vi "RFmx_Cntr_Configure.vi"(7 "Meas_Type":string[](array[string])=["ACP"], 8 "error in (no error)":errorcluster, 10 "RFmx_Parameters":T1={"Default"={"Center_Freq(Hz)"=1150000000.0, "Ref_Level(dBm)"=-10.0, "Span(Hz)"=20000000.0, "RBW(Hz)"=10000.0, "RBW Filter Type"=enum."Gaussian", "Ch_IBW(Hz)"=3840000.0, "Sweep_Time(s)"=0.01, "Num_of_Average"=0, "IQ_Bandwidth(Hz)"=20000000.0}, "ACP_Offset_Freq"=[5000000.0, 10000000.0, 12500000.0], "ACP_Offset_IBW"=[3840000.0, 3840000.0, 3840000.0], "OBW_Percent(%)"=95.0, "TXP_Interval(s)"=0.01, "CCDF_Interval(s)"=0.01, "CCDF_Threshold"=20000000.0, "SFDR_Span(Hz)"=20000000.0, "Harms_RBW(Hz)"=10000.0, "Harms_RBW_Filter"=enum."Gaussian"} {"Harms_RBW(Hz)" format="%.3p"; "TXP_Interval(s)" format="%#_6p"; "SFDR_Span(Hz)" format="%#_6p"; "CCDF_Threshold" format="%#_6p"; "CCDF_Interval(s)" format="%#_6p"; "OBW_Percent(%)" format="%#_6p"; "ACP_Offset_IBW" format="%#_6p"; "ACP_Offset_Freq" format="%#_6p"; "Default"."IQ_Bandwidth(Hz)" format="%#_6p"; "Default"."Num_of_Average" format="%#_6p"; "Default"."Sweep_Time(s)" format="%#_6p"; "Default"."Ch_IBW(Hz)" format="%.3p"; "Default"."RBW(Hz)" format="%.3p"; "Default"."Span(Hz)" format="%.3p"; "Default"."Ref_Level(dBm)" format="%.3p"; "Default"."Center_Freq(Hz)" format="%.3p"}, 11 "Instrument Handle in":refnum<k21>="VST") -> (0 "error out":errorcluster, 3 "Instrument Handle out":refnum<k21>="VST")   [LabVIEW 2014]
uses:
  15_DataManagement/Config_RFmx_Settings.ctl
  <vilib>/RFmx/RFInstr/mx/RFmxInstr.llb/RFmxInstr Build Signal String.vi
  <vilib>/RFmx/SpecAn/mx/RFmxSpecAn.llb/RFmxSpecAn Select Measurement (Single).vi
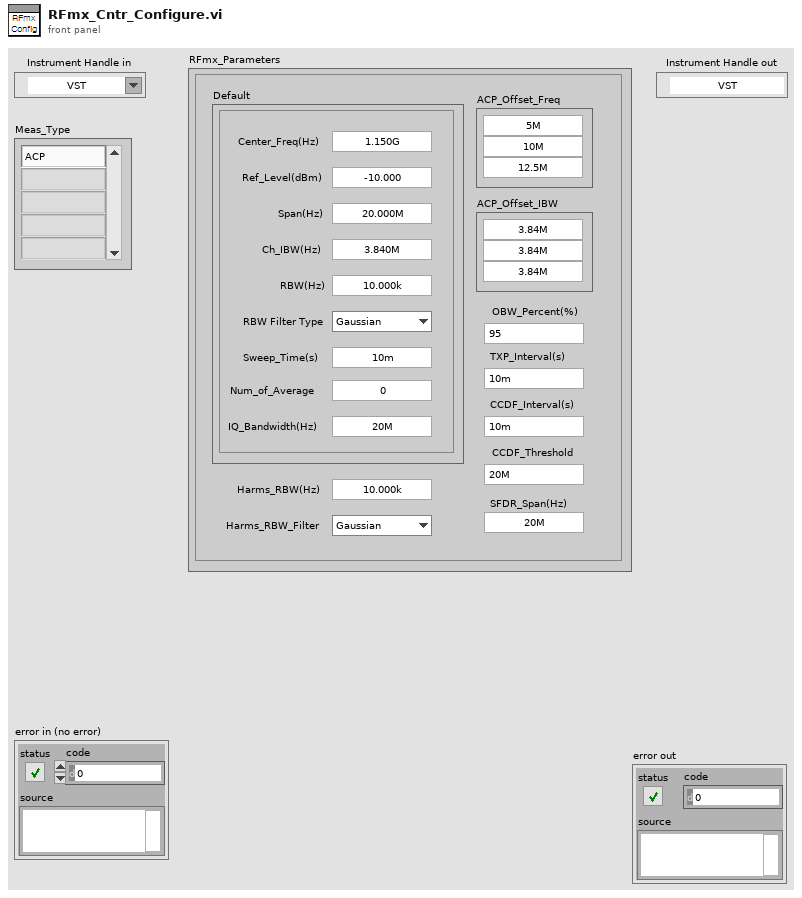
[diagram p1: front panel]
types:
  T1 = typedef "Config_RFmx_Settings.ctl" = cluster{"Default":cluster{"Center_Freq(Hz)":dbl, "Ref_Level(dBm)":dbl, "Span(Hz)":dbl, "RBW(Hz)":dbl, "RBW Filter Type":enum16{"FFT Based", "Gaussian", "Flat", "Synch Tuned - 4", "Synch Tuned - 5"}, "Ch_IBW(Hz)":dbl, "Sweep_Time(s)":dbl, "Num_of_Average":i32, "IQ_Bandwidth(Hz)":dbl}, "ACP_Offset_Freq":dbl[], "ACP_Offset_IBW":dbl[], "OBW_Percent(%)":dbl, "TXP_Interval(s)":dbl, "CCDF_Interval(s)":dbl, "CCDF_Threshold":dbl, "SFDR_Span(Hz)":dbl, "Harms_RBW(Hz)":dbl, "Harms_RBW_Filter":enum16{"FFT Based", "Gaussian", "Flat", "Synch Tuned - 4", "Synch Tuned - 5"}}
  T2 = enum16{"ACP", "CCDF", "CHP", "FCnt", "Harmonics", "OBW", "SEM", "Spectrum", "Spur", "TXP", "AMPM", "DPD", "IQ"}
  T3 = enum16{"FFT Based", "Gaussian", "Flat", "Synch Tuned - 4", "Synch Tuned - 5"}
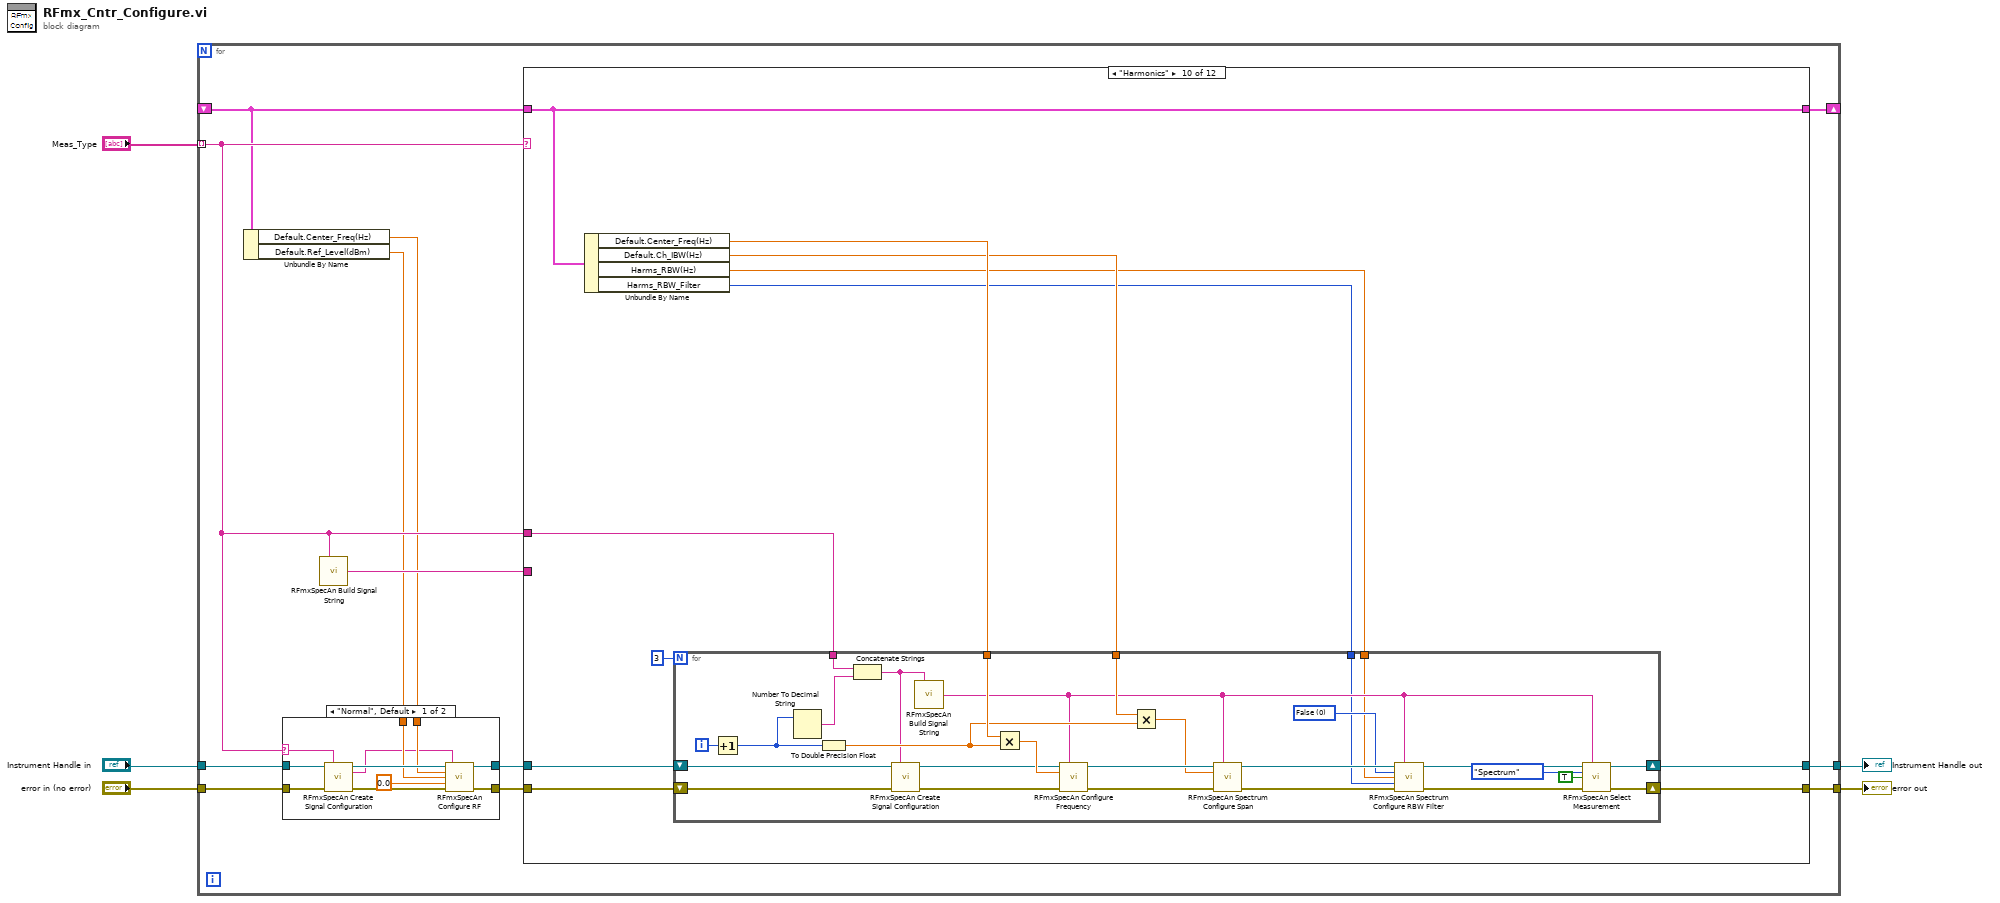
[diagram p0: block diagram]
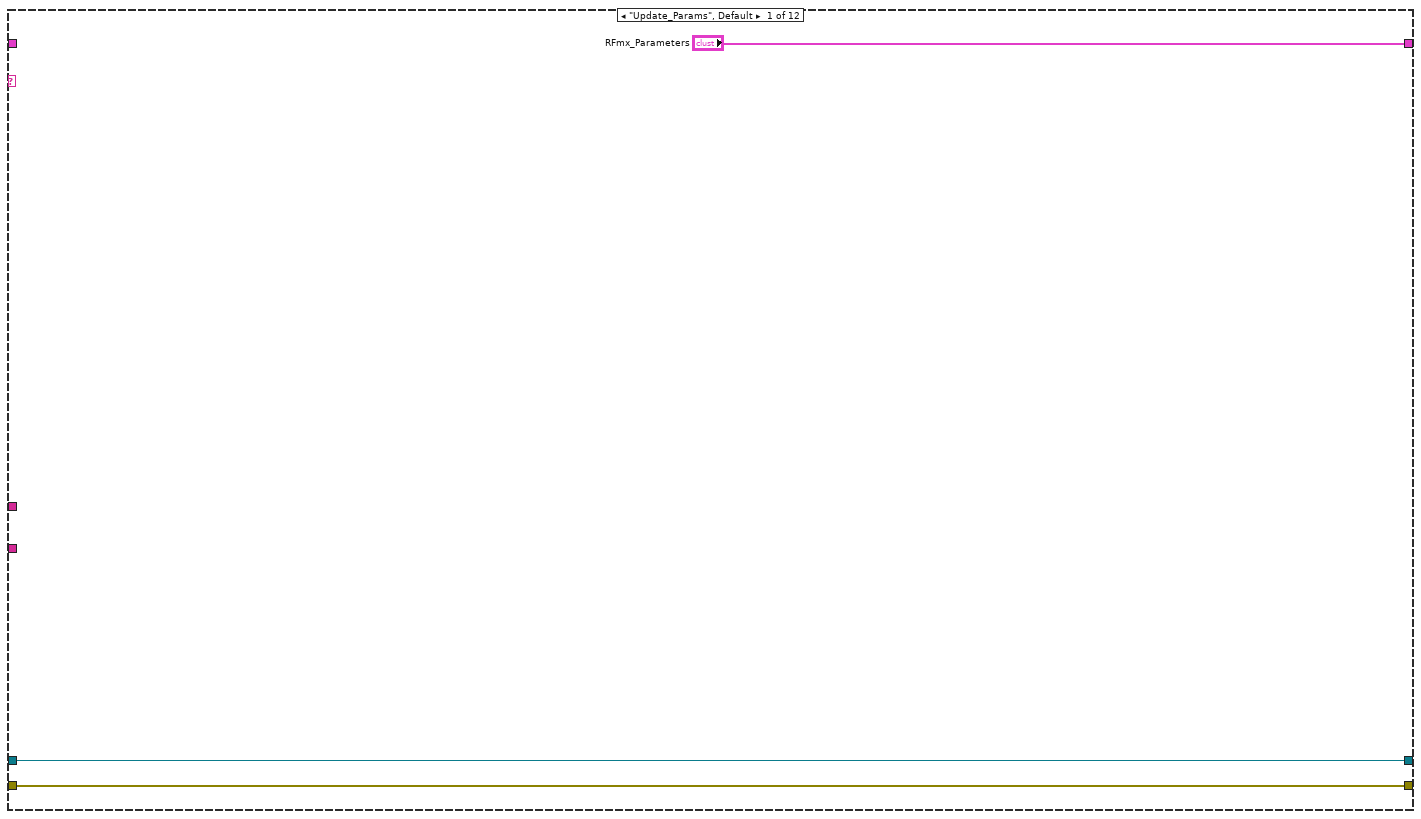
[diagram p3: hidden frame]
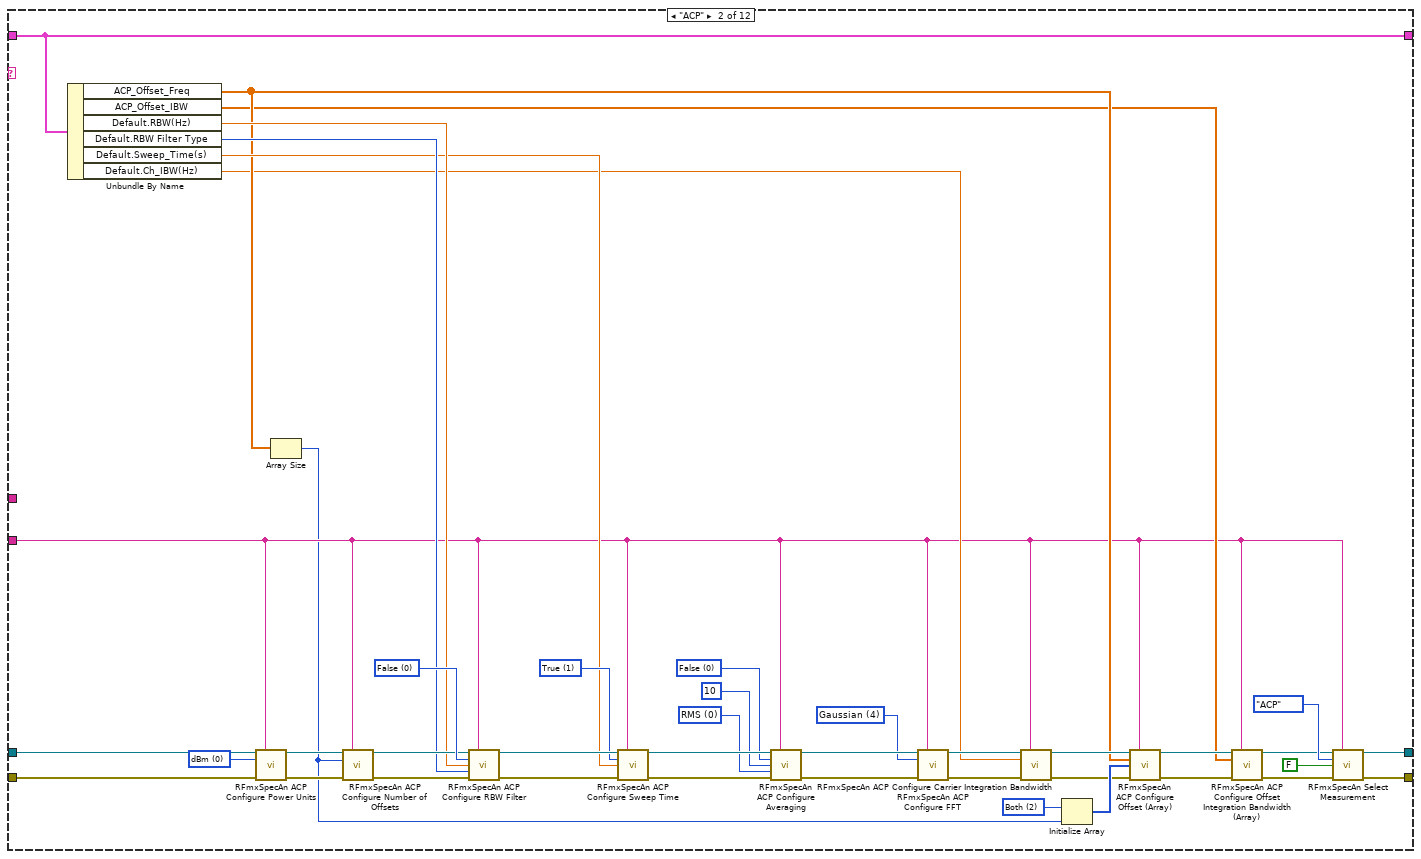
[diagram p4: hidden frame]
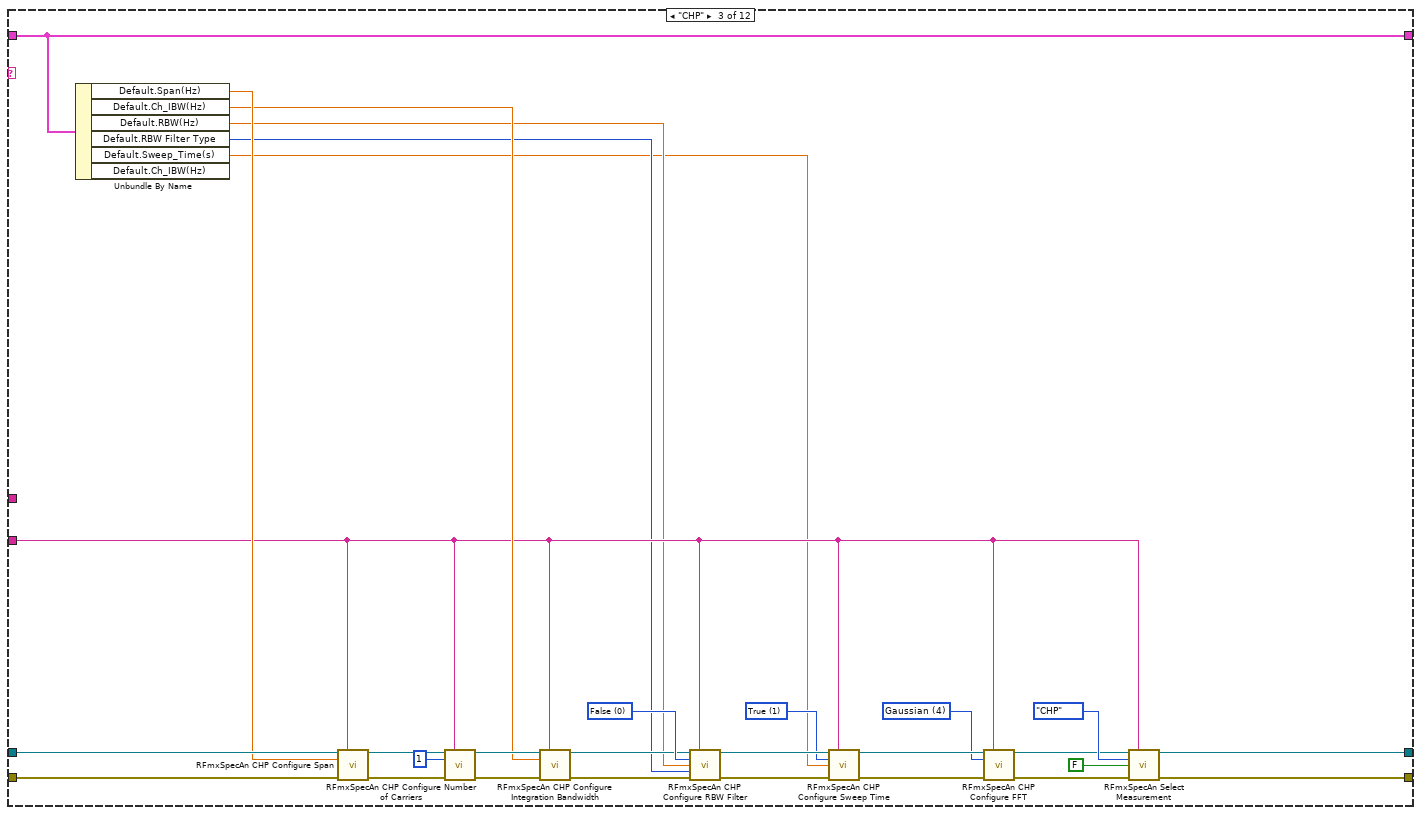
[diagram p5: hidden frame]
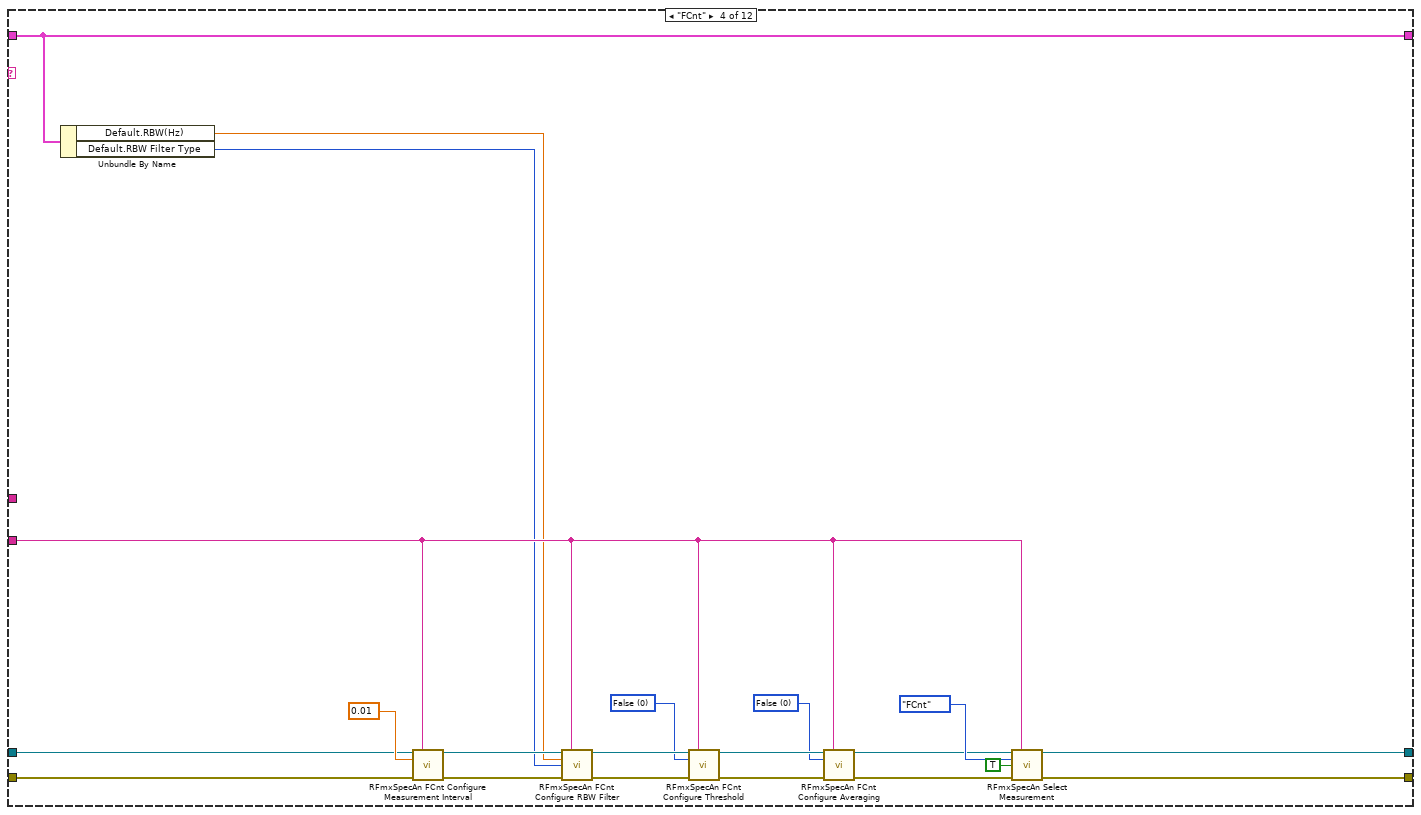
[diagram p6: hidden frame]
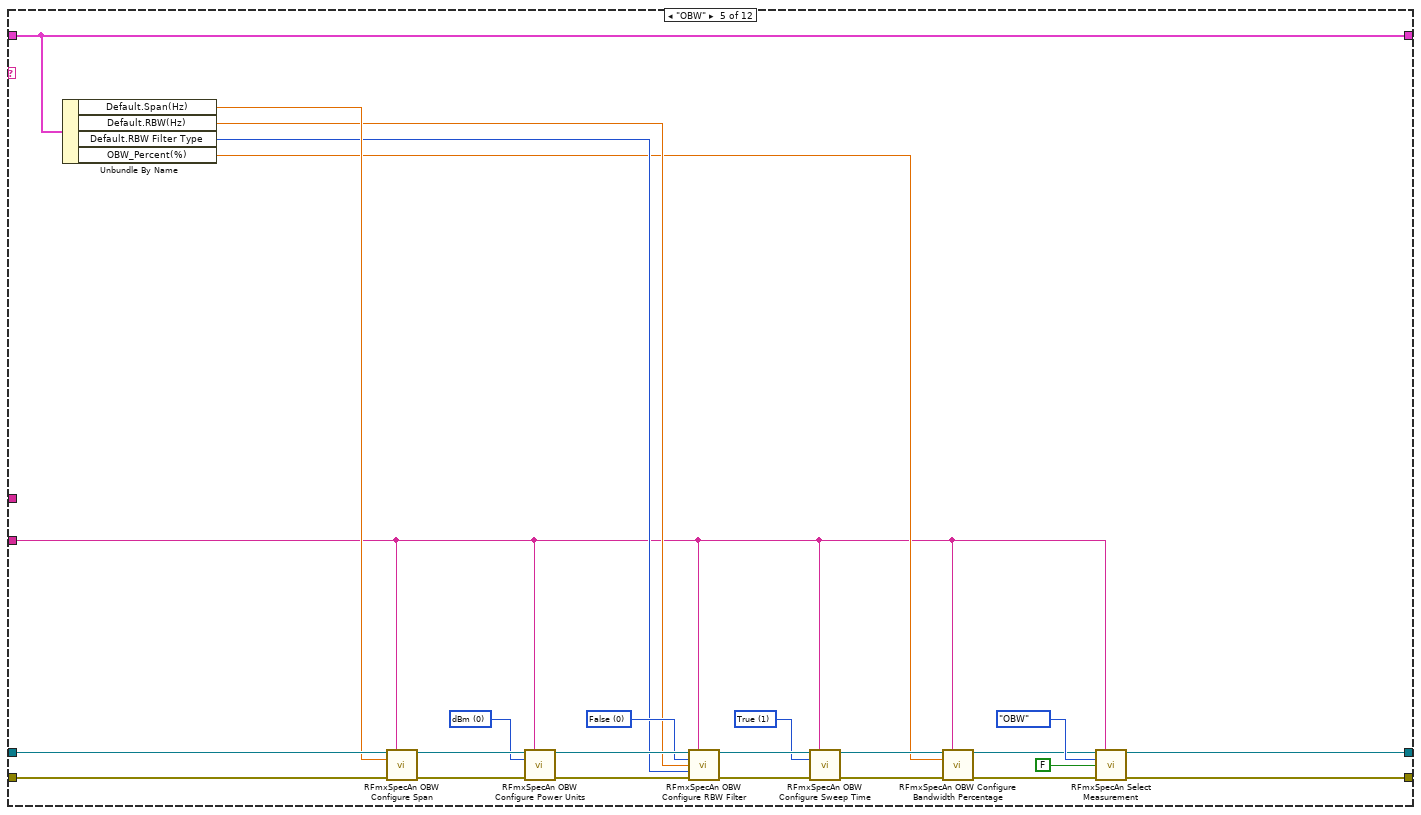
[diagram p7: hidden frame]
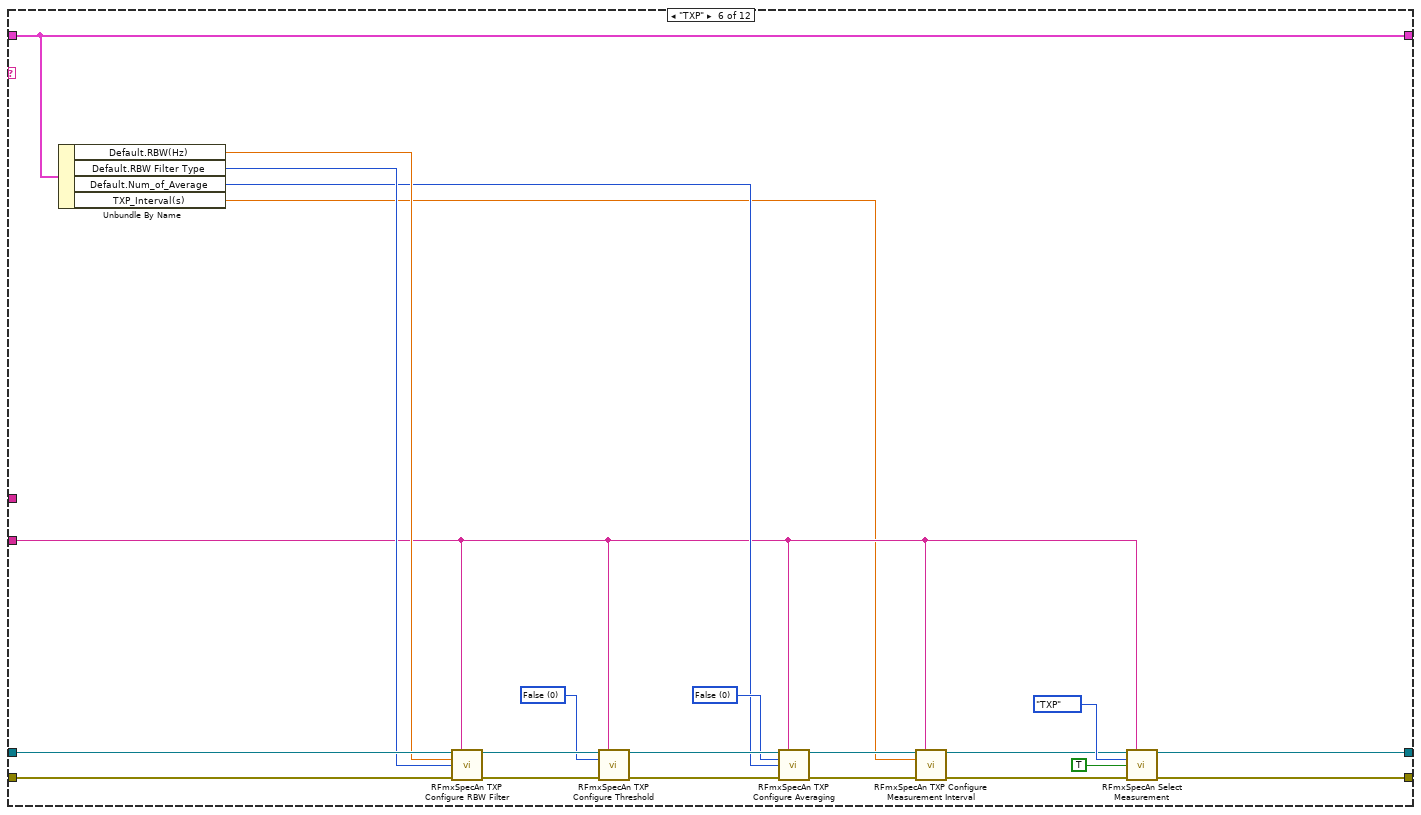
[diagram p8: hidden frame]
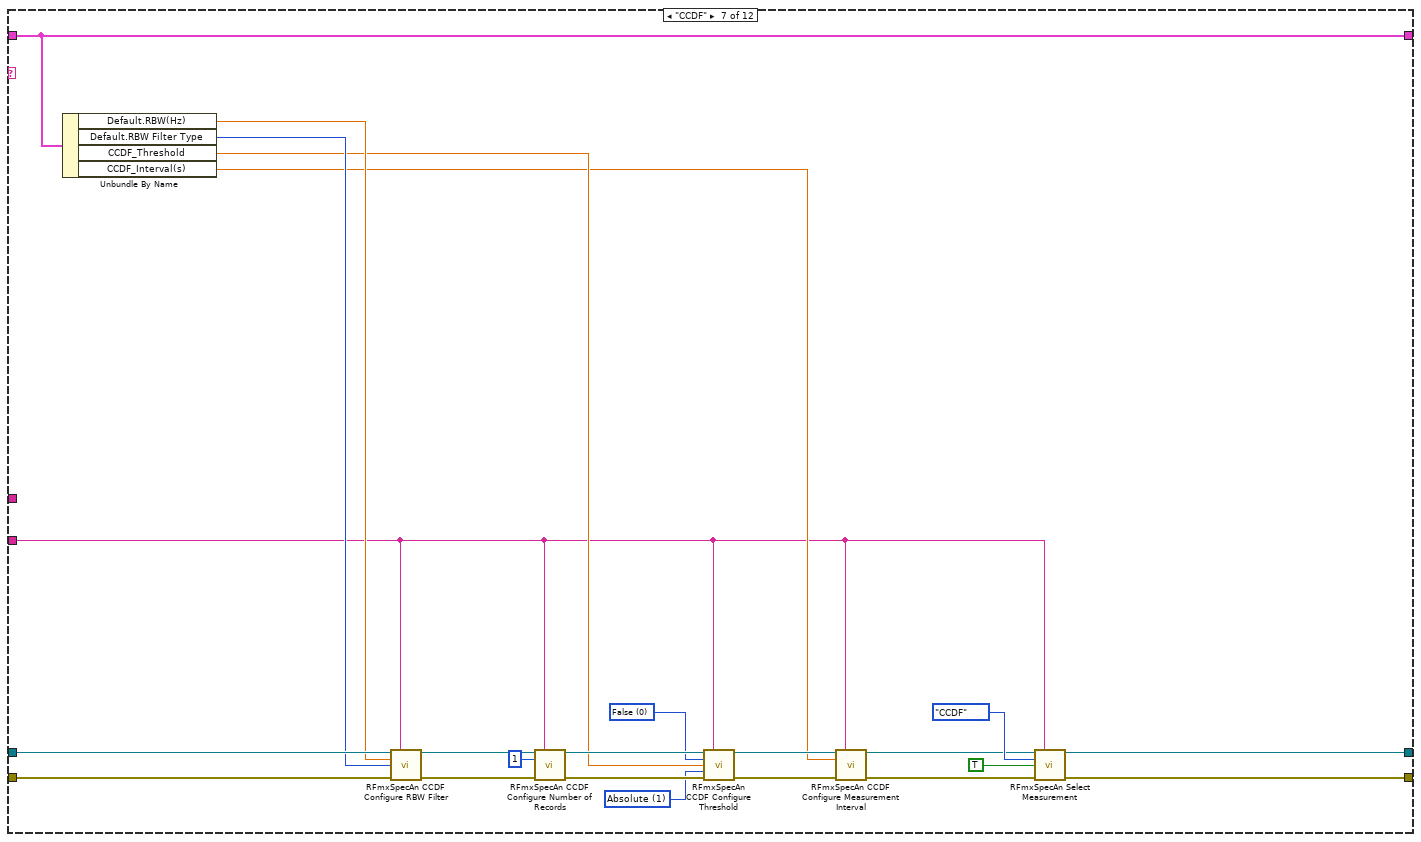
[diagram p9: hidden frame]
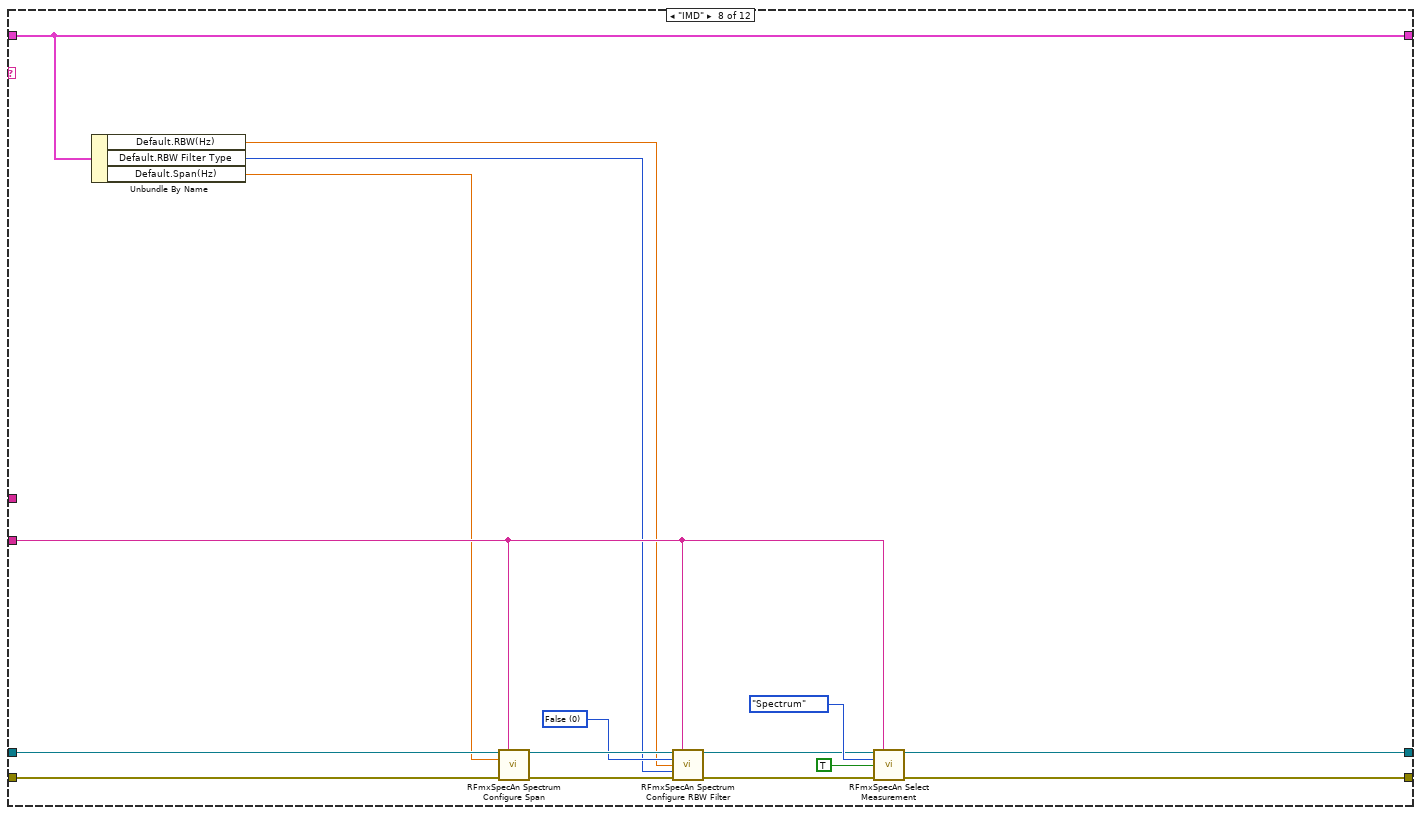
[diagram p10: hidden frame]
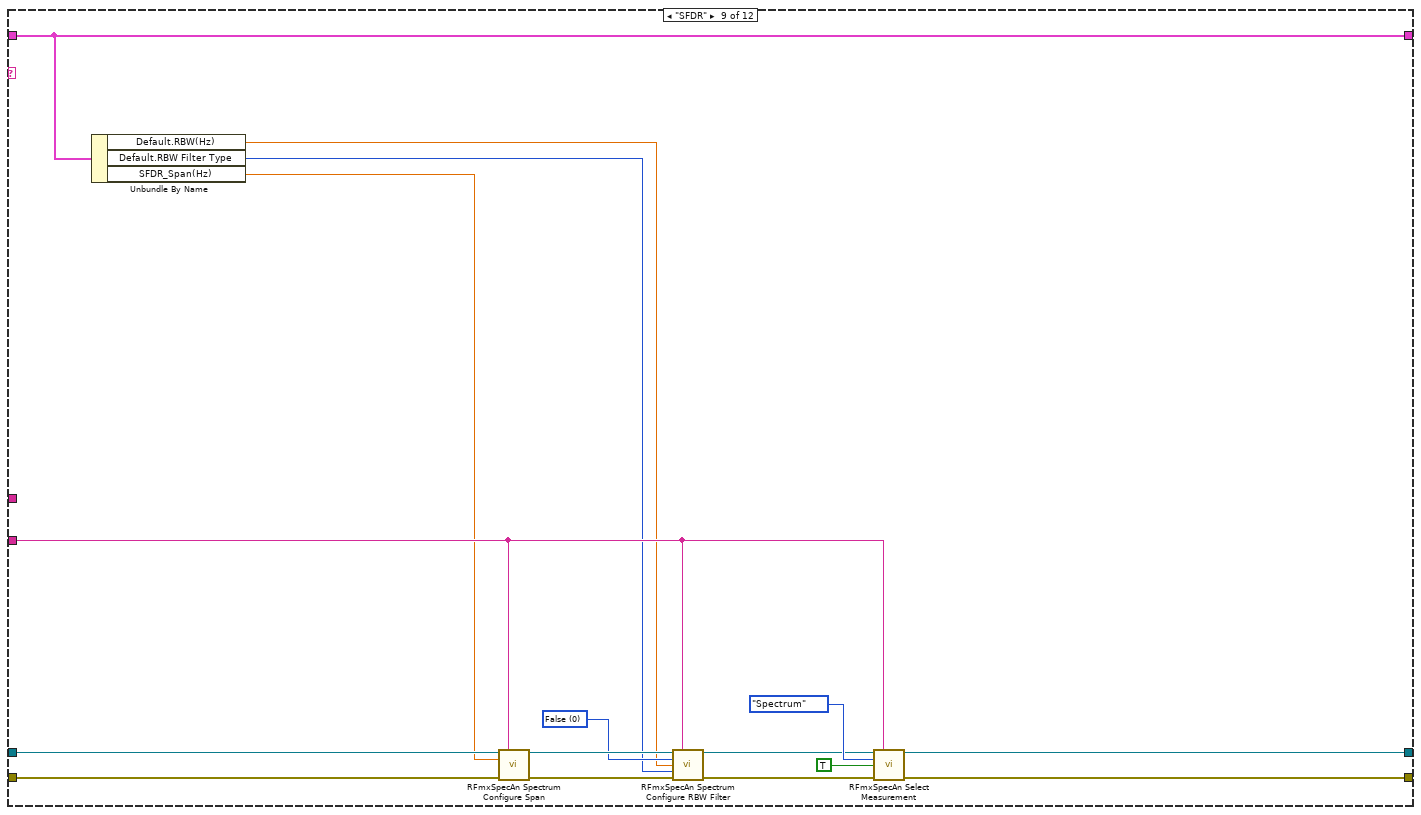
[diagram p11: hidden frame]
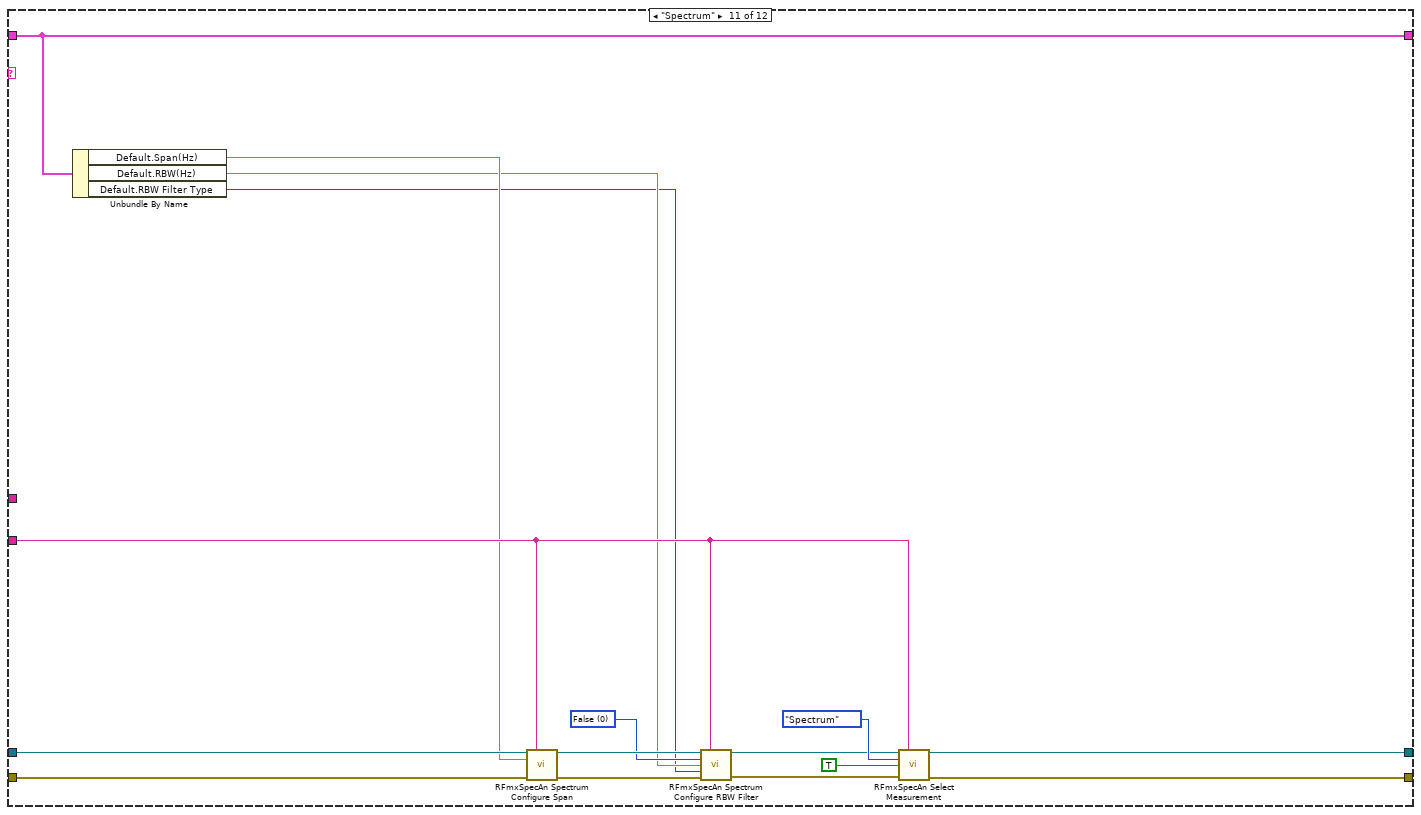
[diagram p12: hidden frame]
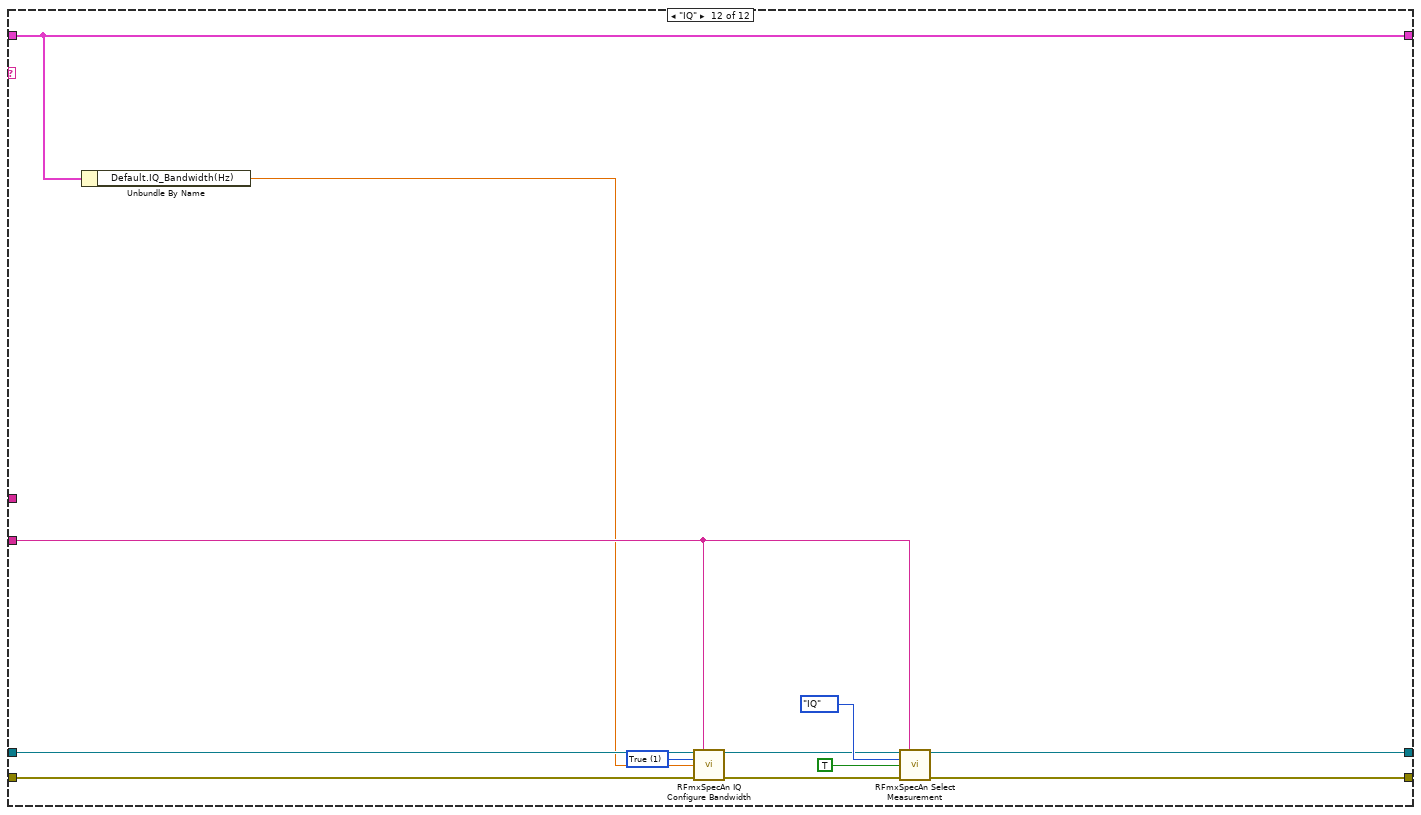
[diagram p13: hidden frame]
diagram:
  n1 = for {
    tunnel: [w17] -> w5
    tunnel: [w16] -> w4
    tunnel: "Meas_Type" -> [w13] mode=indexing
    tunnel: "Instrument Handle in" -> [w15]
    tunnel: "error in (no error)" -> [w14]
    shift-right: [w9] -> _
    shift-left: _ -> [w8]
    n2 = Unbundle By Name(w8) -> ("Default.Center_Freq(Hz)"=w7:dbl, "Default.Ref_Level(dBm)"=w6:dbl)
    n3 = case shown="\"Normal\", Default" w13 {
      selector: w13 -> [w19 _]
      tunnel: w15 -> [w28 w30]
      tunnel: w14 -> [w27 w29]
      tunnel: [w24 w30] -> w11
      tunnel: [w23 w29] -> w10
      tunnel: w6 -> [w21 _]
      tunnel: w7 -> [w20 _]
      frame "Normal", Default {
        n4 = call <vilib>:"RFmxSpecAn Create Signal Configuration.vi"("Instrument Handle In"=w28, "Signal Name"=w19, "error in (no error)"=w27) -> ("Instrument Handle Out"=w25:refnum<k21>, "Selector String Out"=w18:string, "error out"=w22:errorcluster)  [unwired: 10 in]
        n5 = call <vilib>:"RFmxSpecAn Configure RF.vi"("Instrument Handle In"=w25, "Selector String"=w18, "Center Frequency (Hz)"=w20, "Reference Level (dBm)"=w21, "External Attenuation (dB)"=0.0, "error in (no error)"=w22) -> ("Instrument Handle Out"=w24:refnum<k21>, "error out"=w23:errorcluster)  [unwired: 8 in]
      }
      frame "Harmonics" {
      }
    }
    n6 = call <vilib>:"RFmxSpecAn Build Signal String.vi"("Signal Name"=w13) -> ("Selector String"=w12:string)  [unwired: 14 in]
    n7 = case shown="\"Harmonics\"" w13 {
      tunnel: w11 -> [w32 w58 w96 w116 w141 w166 w195 w205 w221 w237 w279 w293]
      tunnel: w10 -> [w31 w57 w95 w115 w140 w165 w194 w204 w220 w236 w278 w292]
      tunnel: [w32 w55 w89 w110 w138 w163 w185 w203 w219 w235 w274 w287] -> w16
      tunnel: [w31 w54 w88 w109 w137 w162 w184 w202 w218 w234 w273 w286] -> w17
      tunnel: w12 -> [_ w36 w81 w111 w128 w152 w173 w201 w217 _ w272 w288]
      tunnel: w13 -> [_ _ _ _ _ _ _ _ _ w233 _ _]
      tunnel: ["RFmx_Parameters" w34 w76 w107 w126 w158 w182 w200 w216 w228 w270 w283] -> w9
      tunnel: w8 -> [_ w34 w76 w107 w126 w158 w182 w200 w216 w228 w270 w283]
      frame "Update_Params", Default {
      }
      frame "ACP" {
        w48 = 2 items=["Neg", "Pos", "Both"] ("Offset Frequency Sideband")
        w63 = 1 items=["False", "True"] ("Sweep Time Auto")
        w64 = 0 items=["RMS", "Log", "Scalar", "Max", "Min", "Vector"] ("Averaging Type")
        w66 = 0 items=["False", "True"] ("Averaging Enabled")
        w67 = 4 items=["None", "Flat Top", "Hanning", "Hamming", "Gaussian", "Blackman", "Blackman-Harris", "Kaiser-Bessel"] ("FFT Window")
        w74 = 0 items=["False", "True"] ("RBW Auto")
        w75 = 0 items=["dBm", "dBm/Hz"] ("Power Units")
        n8 = Unbundle By Name(w34) -> ("ACP_Offset_Freq"=w41:dbl[], "ACP_Offset_IBW"=w39:dbl[], "Default.RBW(Hz)"=w52:dbl, "Default.RBW Filter Type"=w51:T3, "Default.Sweep_Time(s)"=w50:dbl, "Default.Ch_IBW(Hz)"=w40:dbl)
        n9 = call <vilib>:"RFmxSpecAn ACP Configure Power Units.vi"("Instrument Handle In"=w58, "Selector String"=w36, "Power Units"=w75, "error in (no error)"=w57) -> ("Instrument Handle Out"=w62:refnum<k21>, "error out"=w61:errorcluster)  [unwired: 10 in]
        n10 = Array Size(array=w41) -> (size(s)=w35:i32)
        n11 = call <vilib>:"RFmxSpecAn ACP Configure Number of Offsets.vi"("Instrument Handle In"=w62, "Selector String"=w36, "Number of Offsets"=w35, "error in (no error)"=w61) -> ("Instrument Handle Out"=w60:refnum<k21>, "error out"=w59:errorcluster)  [unwired: 10 in]
        n12 = call <vilib>:"RFmxSpecAn ACP Configure RBW Filter.vi"("Instrument Handle In"=w60, "Selector String"=w36, "RBW Auto"=w74, "RBW (Hz)"=w52, "RBW Filter Type"=w51, "error in (no error)"=w59) -> ("Instrument Handle Out"=w73:refnum<k21>, "error out"=w72:errorcluster)  [unwired: 8 in]
        n13 = call <vilib>:"RFmxSpecAn ACP Configure Sweep Time.vi"("Instrument Handle In"=w73, "Selector String"=w36, "Sweep Time Auto"=w63, "Sweep Time Interval (s)"=w50, "error in (no error)"=w72) -> ("Instrument Handle Out"=w71:refnum<k21>, "error out"=w70:errorcluster)  [unwired: 9 in]
        n14 = call <vilib>:"RFmxSpecAn ACP Configure Averaging.vi"("Instrument Handle In"=w71, "Selector String"=w36, "Averaging Enabled"=w66, "Averaging Count"=10, "Averaging Type"=w64, "error in (no error)"=w70) -> ("Instrument Handle Out"=w69:refnum<k21>, "error out"=w68:errorcluster)  [unwired: 8 in]
        n15 = call <vilib>:"RFmxSpecAn ACP Configure FFT.vi"("Instrument Handle In"=w69, "Selector String"=w36, "FFT Window"=w67, "error in (no error)"=w68) -> ("Instrument Handle Out"=w43:refnum<k21>, "error out"=w42:errorcluster)  [unwired: 10 in]
        n16 = call <vilib>:"RFmxSpecAn ACP Configure Carrier Integration Bandwidth.vi"("Instrument Handle In"=w43, "Selector String"=w36, "Integration Bandwidth (Hz)"=w40, "error in (no error)"=w42) -> ("Instrument Handle Out"=w45:refnum<k21>, "error out"=w44:errorcluster)  [unwired: 10 in]
        n17 = Initialize Array(w48, w35) -> (w49:i32[])
        n18 = call <vilib>:"RFmxSpecAn ACP Configure Offset (Array).vi"("Instrument Handle In"=w45, "Selector String"=w36, "Offset Frequency (Hz)"=w41, "Offset Sideband"=w49, "error in (no error)"=w44) -> ("Instrument Handle Out"=w46:refnum<k21>, "error out"=w47:errorcluster)  [unwired: 9 in]
        n19 = call <vilib>:"RFmxSpecAn ACP Configure Offset Integration Bandwidth (Array).vi"("Instrument Handle In"=w46, "Selector String"=w36, "Integration Bandwidth (Hz)"=w39, "error in (no error)"=w47) -> ("Instrument Handle Out"=w38:refnum<k21>, "error out"=w37:errorcluster)  [unwired: 10 in]
        n20 = call-poly <vilib>:"RFmxSpecAn Select Measurement.vi"("Instrument Handle In"=w38, "Selector String"=w36, "Measurement"=T2."ACP", "Enable All Traces"=FALSE, "error in (no error)"=w37) -> ("Instrument Handle Out"=w55:refnum<k21>, "error out"=w54:errorcluster)  [unwired: 9 in]
      }
      frame "CHP" {
        w97 = 4 items=["None", "Flat Top", "Hanning", "Hamming", "Gaussian", "Blackman", "Blackman-Harris", "Kaiser-Bessel"] ("FFT Window")
        w100 = 1 items=["False", "True"] ("Sweep Time Auto")
        w103 = 0 items=["False", "True"] ("RBW Auto")
        n21 = Unbundle By Name(w76) -> ("Default.Span(Hz)"=w85:dbl, "Default.Ch_IBW(Hz)"=w84:dbl, "Default.RBW(Hz)"=w80:dbl, "Default.RBW Filter Type"=w79:T3, "Default.Sweep_Time(s)"=w78:dbl)  [unwired: 1 out]
        n22 = call <vilib>:"RFmxSpecAn CHP Configure Span.vi"("Instrument Handle In"=w96, "Selector String"=w81, "Span (Hz)"=w85, "error in (no error)"=w95) -> ("Instrument Handle Out"=w94:refnum<k21>, "error out"=w93:errorcluster)  [unwired: 10 in]
        n23 = call <vilib>:"RFmxSpecAn CHP Configure Number of Carriers.vi"("Instrument Handle In"=w94, "Selector String"=w81, "Number of Carriers"=1, "error in (no error)"=w93) -> ("Instrument Handle Out"=w87:refnum<k21>, "error out"=w86:errorcluster)  [unwired: 10 in]
        n24 = call <vilib>:"RFmxSpecAn CHP Configure Integration Bandwidth.vi"("Instrument Handle In"=w87, "Selector String"=w81, "Integration Bandwidth (Hz)"=w84, "error in (no error)"=w86) -> ("Instrument Handle Out"=w83:refnum<k21>, "error out"=w82:errorcluster)  [unwired: 10 in]
        n25 = call <vilib>:"RFmxSpecAn CHP Configure RBW Filter.vi"("Instrument Handle In"=w83, "Selector String"=w81, "RBW Auto"=w103, "RBW (Hz)"=w80, "RBW Filter Type"=w79, "error in (no error)"=w82) -> ("Instrument Handle Out"=w102:refnum<k21>, "error out"=w101:errorcluster)  [unwired: 8 in]
        n26 = call <vilib>:"RFmxSpecAn CHP Configure Sweep Time.vi"("Instrument Handle In"=w102, "Selector String"=w81, "Sweep Time Auto"=w100, "Sweep Time Interval (s)"=w78, "error in (no error)"=w101) -> ("Instrument Handle Out"=w99:refnum<k21>, "error out"=w98:errorcluster)  [unwired: 9 in]
        n27 = call <vilib>:"RFmxSpecAn CHP Configure FFT.vi"("Instrument Handle In"=w99, "Selector String"=w81, "FFT Window"=w97, "error in (no error)"=w98) -> ("Instrument Handle Out"=w91:refnum<k21>, "error out"=w90:errorcluster)  [unwired: 10 in]
        n28 = call-poly <vilib>:"RFmxSpecAn Select Measurement.vi"("Instrument Handle In"=w91, "Selector String"=w81, "Measurement"=T2."CHP", "Enable All Traces"=FALSE, "error in (no error)"=w90) -> ("Instrument Handle Out"=w89:refnum<k21>, "error out"=w88:errorcluster)  [unwired: 9 in]
      }
      frame "FCnt" {
        w118 = 0 items=["False", "True"] ("Averaging Enabled")
        w120 = 0 items=["False", "True"] ("Threshold Enabled")
        n29 = Unbundle By Name(w107) -> ("Default.RBW(Hz)"=w106:dbl, "Default.RBW Filter Type"=w105:T3)
        n30 = call <vilib>:"RFmxSpecAn FCnt Configure Measurement Interval.vi"("Instrument Handle In"=w116, "Selector String"=w111, "Measurement Interval (s)"=0.01, "error in (no error)"=w115) -> ("Instrument Handle Out"=w124:refnum<k21>, "error out"=w123:errorcluster)  [unwired: 10 in]
        n31 = call <vilib>:"RFmxSpecAn FCnt Configure RBW Filter.vi"("Instrument Handle In"=w124, "Selector String"=w111, "RBW (Hz)"=w106, "RBW Filter Type"=w105, "error in (no error)"=w123) -> ("Instrument Handle Out"=w122:refnum<k21>, "error out"=w121:errorcluster)  [unwired: 9 in]
        n32 = call <vilib>:"RFmxSpecAn FCnt Configure Threshold.vi"("Instrument Handle In"=w122, "Selector String"=w111, "Threshold Enabled"=w120, "error in (no error)"=w121) -> ("Instrument Handle Out"=w119:refnum<k21>, "error out"=w117:errorcluster)  [unwired: 10 in]
        n33 = call <vilib>:"RFmxSpecAn FCnt Configure Averaging.vi"("Instrument Handle In"=w119, "Selector String"=w111, "Averaging Enabled"=w118, "error in (no error)"=w117) -> ("Instrument Handle Out"=w113:refnum<k21>, "error out"=w112:errorcluster)  [unwired: 10 in]
        n34 = call-poly <vilib>:"RFmxSpecAn Select Measurement.vi"("Instrument Handle In"=w113, "Selector String"=w111, "Measurement"=T2."FCnt", "Enable All Traces"=TRUE, "error in (no error)"=w112) -> ("Instrument Handle Out"=w110:refnum<k21>, "error out"=w109:errorcluster)  [unwired: 9 in]
      }
      frame "OBW" {
        w142 = 1 items=["False", "True"] ("Sweep Time Auto")
        w145 = 0 items=["False", "True"] ("RBW Auto")
        w148 = 0 items=["dBm", "dBm/Hz"] ("Power Units")
        n35 = Unbundle By Name(w126) -> ("Default.Span(Hz)"=w132:dbl, "Default.RBW(Hz)"=w131:dbl, "Default.RBW Filter Type"=w130:T3, "OBW_Percent(%)"=w129:dbl)
        n36 = call <vilib>:"RFmxSpecAn OBW Configure Span.vi"("Instrument Handle In"=w141, "Selector String"=w128, "Span (Hz)"=w132, "error in (no error)"=w140) -> ("Instrument Handle Out"=w150:refnum<k21>, "error out"=w149:errorcluster)  [unwired: 10 in]
        n37 = call <vilib>:"RFmxSpecAn OBW Configure Power Units.vi"("Instrument Handle In"=w150, "Selector String"=w128, "Power Units"=w148, "error in (no error)"=w149) -> ("Instrument Handle Out"=w147:refnum<k21>, "error out"=w146:errorcluster)  [unwired: 10 in]
        n38 = call <vilib>:"RFmxSpecAn OBW Configure RBW Filter.vi"("Instrument Handle In"=w147, "Selector String"=w128, "RBW Auto"=w145, "RBW (Hz)"=w131, "RBW Filter Type"=w130, "error in (no error)"=w146) -> ("Instrument Handle Out"=w144:refnum<k21>, "error out"=w143:errorcluster)  [unwired: 8 in]
        n39 = call <vilib>:"RFmxSpecAn OBW Configure Sweep Time.vi"("Instrument Handle In"=w144, "Selector String"=w128, "Sweep Time Auto"=w142, "error in (no error)"=w143) -> ("Instrument Handle Out"=w136:refnum<k21>, "error out"=w135:errorcluster)  [unwired: 10 in]
        n40 = call <vilib>:"RFmxSpecAn OBW Configure Bandwidth Percentage.vi"("Instrument Handle In"=w136, "Selector String"=w128, "Bandwidth Percentage (%)"=w129, "error in (no error)"=w135) -> ("Instrument Handle Out"=w134:refnum<k21>, "error out"=w133:errorcluster)  [unwired: 10 in]
        n41 = call-poly <vilib>:"RFmxSpecAn Select Measurement.vi"("Instrument Handle In"=w134, "Selector String"=w128, "Measurement"=T2."OBW", "Enable All Traces"=FALSE, "error in (no error)"=w133) -> ("Instrument Handle Out"=w138:refnum<k21>, "error out"=w137:errorcluster)  [unwired: 9 in]
      }
      frame "TXP" {
        w167 = 0 items=["False", "True"] ("Averaging Enabled")
        w171 = 0 items=["False", "True"] ("Threshold Enabled")
        n42 = Unbundle By Name(w158) -> ("Default.RBW(Hz)"=w160:dbl, "Default.RBW Filter Type"=w159:T3, "Default.Num_of_Average"=w157:i32, "TXP_Interval(s)"=w151:dbl)
        n43 = call <vilib>:"RFmxSpecAn TXP Configure RBW Filter.vi"("Instrument Handle In"=w166, "Selector String"=w152, "RBW (Hz)"=w160, "RBW Filter Type"=w159, "error in (no error)"=w165) -> ("Instrument Handle Out"=w172:refnum<k21>, "error out"=w170:errorcluster)  [unwired: 9 in]
        n44 = call <vilib>:"RFmxSpecAn TXP Configure Threshold.vi"("Instrument Handle In"=w172, "Selector String"=w152, "Threshold Enabled"=w171, "error in (no error)"=w170) -> ("Instrument Handle Out"=w169:refnum<k21>, "error out"=w168:errorcluster)  [unwired: 10 in]
        n45 = call <vilib>:"RFmxSpecAn TXP Configure Averaging.vi"("Instrument Handle In"=w169, "Selector String"=w152, "Averaging Enabled"=w167, "Averaging Count"=w157, "error in (no error)"=w168) -> ("Instrument Handle Out"=w156:refnum<k21>, "error out"=w155:errorcluster)  [unwired: 9 in]
        n46 = call <vilib>:"RFmxSpecAn TXP Configure Measurement Interval.vi"("Instrument Handle In"=w156, "Selector String"=w152, "Measurement Interval (s)"=w151, "error in (no error)"=w155) -> ("Instrument Handle Out"=w154:refnum<k21>, "error out"=w153:errorcluster)  [unwired: 10 in]
        n47 = call-poly <vilib>:"RFmxSpecAn Select Measurement.vi"("Instrument Handle In"=w154, "Selector String"=w152, "Measurement"=T2."TXP", "Enable All Traces"=TRUE, "error in (no error)"=w153) -> ("Instrument Handle Out"=w163:refnum<k21>, "error out"=w162:errorcluster)  [unwired: 9 in]
      }
      frame "CCDF" {
        w187 = 1 items=["Relative", "Absolute"] ("Threshold Type")
        w188 = 0 items=["False", "True"] ("Threshold Enabled")
        n48 = Unbundle By Name(w182) -> ("Default.RBW(Hz)"=w181:dbl, "Default.RBW Filter Type"=w180:T3, "CCDF_Threshold"=w179:dbl, "CCDF_Interval(s)"=w176:dbl)
        n49 = call <vilib>:"RFmxSpecAn CCDF Configure RBW Filter.vi"("Instrument Handle In"=w195, "Selector String"=w173, "RBW (Hz)"=w181, "RBW Filter Type"=w180, "error in (no error)"=w194) -> ("Instrument Handle Out"=w193:refnum<k21>, "error out"=w192:errorcluster)  [unwired: 9 in]
        n50 = call <vilib>:"RFmxSpecAn CCDF Configure Number of Records.vi"("Instrument Handle In"=w193, "Selector String"=w173, "Number of Records"=1, "error in (no error)"=w192) -> ("Instrument Handle Out"=w191:refnum<k21>, "error out"=w190:errorcluster)  [unwired: 10 in]
        n51 = call <vilib>:"RFmxSpecAn CCDF Configure Threshold.vi"("Instrument Handle In"=w191, "Selector String"=w173, "Threshold Enabled"=w188, "Threshold Level (dB or dBm)"=w179, "Threshold Type"=w187, "error in (no error)"=w190) -> ("Instrument Handle Out"=w178:refnum<k21>, "error out"=w177:errorcluster)  [unwired: 8 in]
        n52 = call <vilib>:"RFmxSpecAn CCDF Configure Measurement Interval.vi"("Instrument Handle In"=w178, "Selector String"=w173, "Measurement Interval (s)"=w176, "error in (no error)"=w177) -> ("Instrument Handle Out"=w175:refnum<k21>, "error out"=w174:errorcluster)  [unwired: 10 in]
        n53 = call-poly <vilib>:"RFmxSpecAn Select Measurement.vi"("Instrument Handle In"=w175, "Selector String"=w173, "Measurement"=T2."CCDF", "Enable All Traces"=TRUE, "error in (no error)"=w174) -> ("Instrument Handle Out"=w185:refnum<k21>, "error out"=w184:errorcluster)  [unwired: 9 in]
      }
      frame "IMD" {
        w209 = 0 items=["False", "True"] ("RBW Auto")
        n54 = Unbundle By Name(w200) -> ("Default.RBW(Hz)"=w199:dbl, "Default.RBW Filter Type"=w198:T3, "Default.Span(Hz)"=w196:dbl)
        n55 = call <vilib>:"RFmxSpecAn Spectrum Configure Span.vi"("Instrument Handle In"=w205, "Selector String"=w201, "Span (Hz)"=w196, "error in (no error)"=w204) -> ("Instrument Handle Out"=w211:refnum<k21>, "error out"=w210:errorcluster)  [unwired: 10 in]
        n56 = call <vilib>:"RFmxSpecAn Spectrum Configure RBW Filter.vi"("Instrument Handle In"=w211, "Selector String"=w201, "RBW Auto"=w209, "RBW (Hz)"=w199, "RBW Filter Type"=w198, "error in (no error)"=w210) -> ("Instrument Handle Out"=w207:refnum<k21>, "error out"=w206:errorcluster)  [unwired: 8 in]
        n57 = call-poly <vilib>:"RFmxSpecAn Select Measurement.vi"("Instrument Handle In"=w207, "Selector String"=w201, "Measurement"=T2."Spectrum", "Enable All Traces"=TRUE, "error in (no error)"=w206) -> ("Instrument Handle Out"=w203:refnum<k21>, "error out"=w202:errorcluster)  [unwired: 9 in]
      }
      frame "SFDR" {
        w225 = 0 items=["False", "True"] ("RBW Auto")
        n58 = Unbundle By Name(w216) -> ("Default.RBW(Hz)"=w215:dbl, "Default.RBW Filter Type"=w214:T3, "SFDR_Span(Hz)"=w212:dbl)
        n59 = call <vilib>:"RFmxSpecAn Spectrum Configure Span.vi"("Instrument Handle In"=w221, "Selector String"=w217, "Span (Hz)"=w212, "error in (no error)"=w220) -> ("Instrument Handle Out"=w227:refnum<k21>, "error out"=w226:errorcluster)  [unwired: 10 in]
        n60 = call <vilib>:"RFmxSpecAn Spectrum Configure RBW Filter.vi"("Instrument Handle In"=w227, "Selector String"=w217, "RBW Auto"=w225, "RBW (Hz)"=w215, "RBW Filter Type"=w214, "error in (no error)"=w226) -> ("Instrument Handle Out"=w223:refnum<k21>, "error out"=w222:errorcluster)  [unwired: 8 in]
        n61 = call-poly <vilib>:"RFmxSpecAn Select Measurement.vi"("Instrument Handle In"=w223, "Selector String"=w217, "Measurement"=T2."Spectrum", "Enable All Traces"=TRUE, "error in (no error)"=w222) -> ("Instrument Handle Out"=w219:refnum<k21>, "error out"=w218:errorcluster)  [unwired: 9 in]
      }
      frame "Harmonics" {
        n62 = Unbundle By Name(w228) -> ("Default.Center_Freq(Hz)"=w232:dbl, "Default.Ch_IBW(Hz)"=w231:dbl, "Harms_RBW(Hz)"=w230:dbl, "Harms_RBW_Filter"=w229:T3)
        n63 = for {
          N: 3 -> [_]
          shift-right: [w247] -> w235
          shift-left: w237 -> [w255]
          shift-right: [w246] -> w234
          shift-left: w236 -> [w254]
          tunnel: w232 -> [w261]
          tunnel: w231 -> [w260]
          tunnel: w233 -> [w244]
          tunnel: w230 -> [w240]
          tunnel: w229 -> [w239]
          i -> [w242]
          w257 = 0 items=["False", "True"] ("RBW Auto")
          n64 = Increment(x=w242) -> (x+1=w241:i32)
          n65 = Number To Decimal String(number=w241) -> (decimal integer string=w256:string)  [unwired: 1 in]
          n66 = To Double Precision Float(number=w241) -> (double precision float=w259:dbl)
          n67 = Concatenate Strings(w244, w256) -> (w253:string)
          n68 = call <vilib>:"RFmxSpecAn Create Signal Configuration.vi"("Instrument Handle In"=w255, "Signal Name"=w253, "error in (no error)"=w254) -> ("Instrument Handle Out"=w252:refnum<k21>, "error out"=w251:errorcluster)  [unwired: 10 in, 1 out]
          n69 = call <vilib>:"RFmxSpecAn Build Signal String.vi"("Signal Name"=w253) -> ("Selector String"=w245:string)  [unwired: 14 in]
          n70 = Multiply(x=w261, y=w259) -> (x*y=w262:dbl)
          n71 = call <vilib>:"RFmxSpecAn Configure Frequency.vi"("Instrument Handle In"=w252, "Selector String"=w245, "Center Frequency (Hz)"=w262, "error in (no error)"=w251) -> ("Instrument Handle Out"=w266:refnum<k21>, "error out"=w265:errorcluster)  [unwired: 10 in]
          n72 = Multiply(x=w260, y=w259) -> (x*y=w258:dbl)
          n73 = call <vilib>:"RFmxSpecAn Spectrum Configure Span.vi"("Instrument Handle In"=w266, "Selector String"=w245, "Span (Hz)"=w258, "error in (no error)"=w265) -> ("Instrument Handle Out"=w264:refnum<k21>, "error out"=w263:errorcluster)  [unwired: 10 in]
          n74 = call <vilib>:"RFmxSpecAn Spectrum Configure RBW Filter.vi"("Instrument Handle In"=w264, "Selector String"=w245, "RBW Auto"=w257, "RBW (Hz)"=w240, "RBW Filter Type"=w239, "error in (no error)"=w263) -> ("Instrument Handle Out"=w250:refnum<k21>, "error out"=w249:errorcluster)  [unwired: 8 in]
          n75 = call-poly <vilib>:"RFmxSpecAn Select Measurement.vi"("Instrument Handle In"=w250, "Selector String"=w245, "Measurement"=T2."Spectrum", "Enable All Traces"=TRUE, "error in (no error)"=w249) -> ("Instrument Handle Out"=w247:refnum<k21>, "error out"=w246:errorcluster)  [unwired: 9 in]
        }
      }
      frame "Spectrum" {
        w280 = 0 items=["False", "True"] ("RBW Auto")
        n76 = Unbundle By Name(w270) -> ("Default.Span(Hz)"=w269:dbl, "Default.RBW(Hz)"=w268:dbl, "Default.RBW Filter Type"=w267:T3)
        n77 = call <vilib>:"RFmxSpecAn Spectrum Configure Span.vi"("Instrument Handle In"=w279, "Selector String"=w272, "Span (Hz)"=w269, "error in (no error)"=w278) -> ("Instrument Handle Out"=w282:refnum<k21>, "error out"=w281:errorcluster)  [unwired: 10 in]
        n78 = call <vilib>:"RFmxSpecAn Spectrum Configure RBW Filter.vi"("Instrument Handle In"=w282, "Selector String"=w272, "RBW Auto"=w280, "RBW (Hz)"=w268, "RBW Filter Type"=w267, "error in (no error)"=w281) -> ("Instrument Handle Out"=w276:refnum<k21>, "error out"=w275:errorcluster)  [unwired: 8 in]
        n79 = call-poly <vilib>:"RFmxSpecAn Select Measurement.vi"("Instrument Handle In"=w276, "Selector String"=w272, "Measurement"=T2."Spectrum", "Enable All Traces"=TRUE, "error in (no error)"=w275) -> ("Instrument Handle Out"=w274:refnum<k21>, "error out"=w273:errorcluster)  [unwired: 9 in]
      }
      frame "IQ" {
        w294 = 1 items=["False", "True"] ("Bandwidth Auto")
        n80 = Unbundle By Name(w283) -> ("Default.IQ_Bandwidth(Hz)"=w284:dbl)
        n81 = call <vilib>:"RFmxSpecAn IQ Configure Bandwidth.vi"("Instrument Handle In"=w293, "Selector String"=w288, "Bandwidth Auto"=w294, "Bandwidth (Hz)"=w284, "error in (no error)"=w292) -> ("Instrument Handle Out"=w290:refnum<k21>, "error out"=w289:errorcluster)  [unwired: 9 in]
        n82 = call-poly <vilib>:"RFmxSpecAn Select Measurement.vi"("Instrument Handle In"=w290, "Selector String"=w288, "Measurement"=T2."IQ", "Enable All Traces"=TRUE, "error in (no error)"=w289) -> ("Instrument Handle Out"=w287:refnum<k21>, "error out"=w286:errorcluster)  [unwired: 9 in]
      }
    }
  }
  "Instrument Handle out" <- w4
  "error out" <- w5
